vi "testscale.vi"() -> ()   [LabVIEW 2011]
panel:
  out "XY Graph":cluster{dbl[], dbl[]}[](graph)
  out "Motor Value":dbl
  in  "stop":bool
  out "ScaledToPercentRange":dbl
  in  "RawValue":i8(slide)=50 scale=-127.0..127.0
  in  "Scaler":i8=127
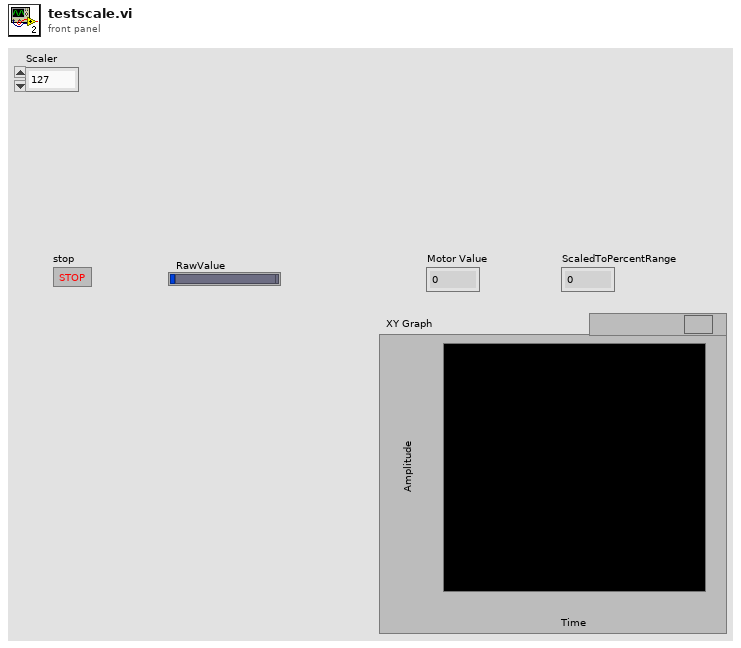
[diagram p1: front panel]
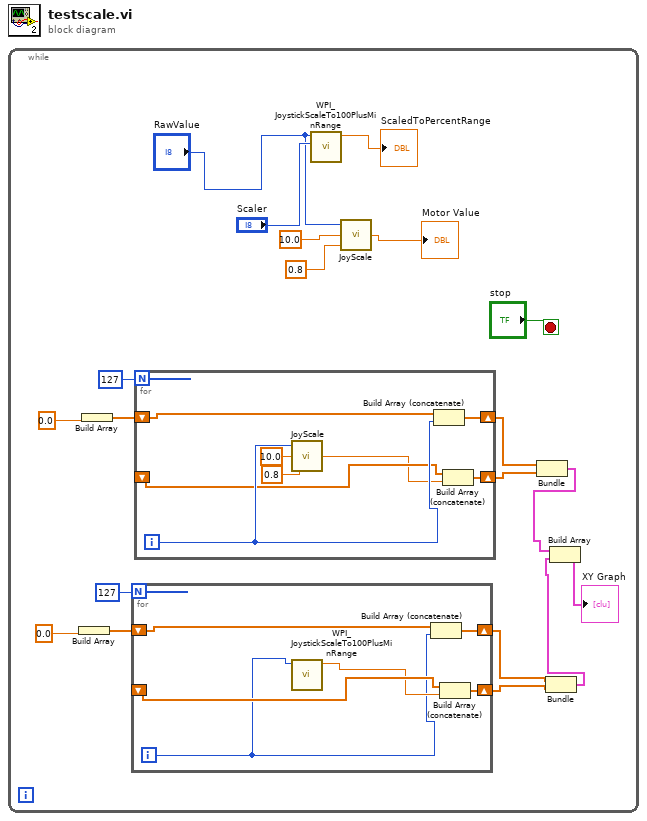
[diagram p0: block diagram]
diagram:
  n1 = while {
    stop <- "stop" stop-if-true
    n2 = Build Array(0.0 ("element")) -> (w6:dbl[])
    n3 = Build Array(0.0 ("element")) -> (w15:dbl[])
    n4 = for {
      N: 127 -> [_]
      shift-right: [w26] -> w5
      shift-left: w6 -> [w25]
      shift-right: [w24] -> w4
      shift-left: _ -> [w23]
      i -> [w21]
      n5 = call <vilib>:"WPI_JoystickScaleTo100PlusMinRange.vi"("RawValue"=w21) -> ("ScaledToPercentRange"=w22:dbl)  [unwired: 1 in, 9 out]
      n6 = Build Array (concatenate)(w25, w21) -> (w26:dbl[])
      n7 = Build Array (concatenate)(w23, w22) -> (w24:dbl[])
    }
    n8 = for {
      N: 127 -> [_]
      shift-right: [w34] -> w14
      shift-left: w15 -> [w33]
      shift-right: [w29] -> w13
      shift-left: _ -> [w28]
      i -> [w32]
      n9 = call "JoyScale.vi"("Max Power"=0.8, "DeadZone"=10.0, "JoyValue"=w32) -> ("Motor Value"=w27:dbl)
      n10 = Build Array (concatenate)(w33, w32) -> (w34:dbl[])
      n11 = Build Array (concatenate)(w28, w27) -> (w29:dbl[])
    }
    n12 = call <vilib>:"WPI_JoystickScaleTo100PlusMinRange.vi"("Scaler"="Scaler", "RawValue"="RawValue") -> ("ScaledToPercentRange"=→"ScaledToPercentRange":dbl)  [unwired: 9 out]
    n13 = call "JoyScale.vi"("Max Power"=0.8, "DeadZone"=10.0, "JoyValue"="RawValue") -> ("Motor Value"=→"Motor Value":dbl)
    n14 = Bundle(w14, w13) -> (w3:cluster{dbl[], dbl[]})  [unwired: 1 in]
    n15 = Bundle(w5, w4) -> (w2:cluster{dbl[], dbl[]})  [unwired: 1 in]
    n16 = Build Array(w3, w2) -> (→"XY Graph":cluster{dbl[], dbl[]}[])
  }
